vi "GPIB Diag.vi"() -> ()   [LabVIEW 2011]
panel:
  in  "frequency (1E+3)":dbl=1000.0 format="%.2p"
  in  "amplitude (2.00)":dbl=2.0 format="%.2p"
  in  "waveform (sine)":i32(ring)=1 items=["Sine"=1, "Square"=2, "Triangle"=3, "Ramp Up"=4, "Noise"=1001]
  out "firmware revision":string
  out "instrument driver revision":string
  in  "resource name (\"GPIB::14::INSTR\")":refnum<k15>="\"GPIB::14::INSTR\""
  # "Select the correct device from the list after refreshing your GPIB Line, then press run.\n\nAlso try setting some function characteristics and see if it follows instructions."
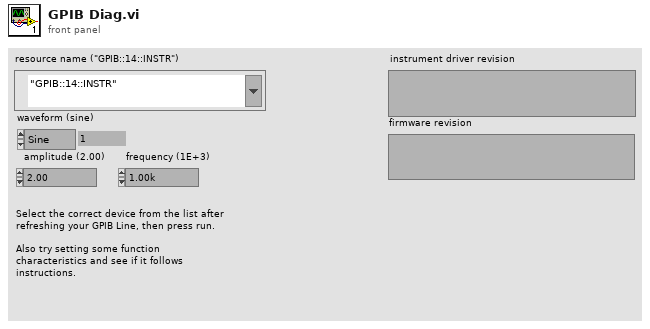
[diagram p1: front panel]
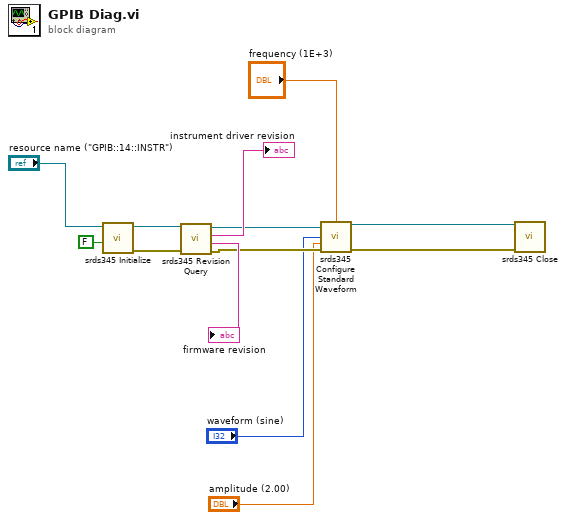
[diagram p0: block diagram]
diagram:
  n1 = call <instrlib>:"srds345 Initialize.vi"("reset device (true)"=FALSE, "resource name (\"GPIB::14::INSTR\")"="resource name (\"GPIB::14::INSTR\")") -> ("error out"=w12:errorcluster, "instrument handle out"=w11:refnum<k15>)  [unwired: 8 in]
  n2 = call <instrlib>:"srds345 Revision Query.vi"("error in (no error)"=w12, "instrument handle"=w11) -> ("error out"=w8:errorcluster, "firmware revision"=→"firmware revision":string, "instrument driver revision"=→"instrument driver revision":string, "instrument handle out"=w7:refnum<k15>)  [unwired: 6 in]
  n3 = call <instrlib>:"srds345 Configure Standard Waveform.vi"("instrument handle"=w7, "frequency (1E+3)"="frequency (1E+3)", "waveform (sine)"="waveform (sine)", "amplitude (2.00)"="amplitude (2.00)", "error in (no error)"=w8) -> ("instrument handle out"=w3:refnum<k15>, "error out"=w4:errorcluster)  [unwired: 9 in]
  n4 = call <instrlib>:"srds345 Close.vi"("error in (no error)"=w4, "instrument handle"=w3) -> ()  [unwired: 9 in, 1 out]
